vi "Untitled 1.vi"() -> ()   [LabVIEW 2018]
panel:
  out "error out":errorcluster
  out "Image Display":T1(plugin-control)
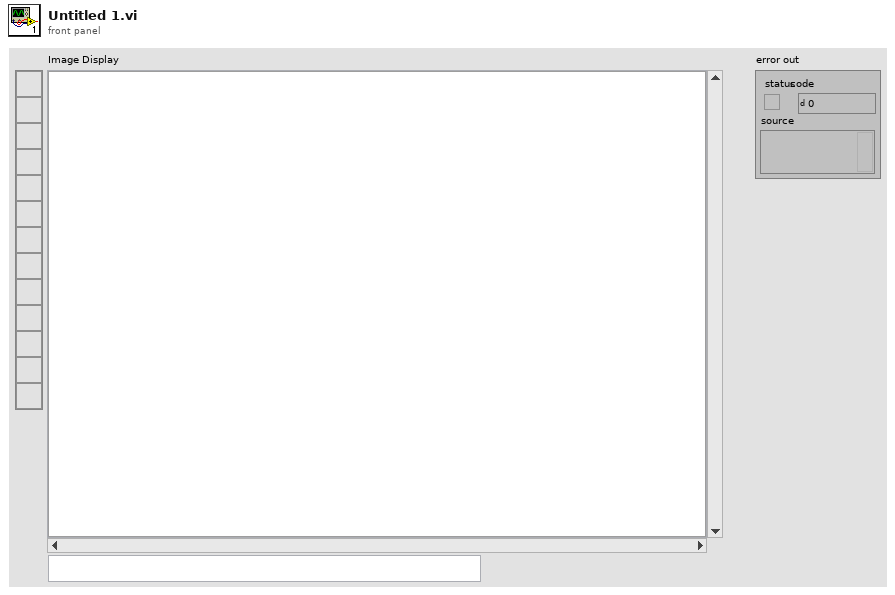
[diagram p1: front panel]
types:
  T1 = typedef "IMAQ Image.ctl" = refnum<image>
  T2 = typedef "Image Type" = u32
  T3 = typedef "imagedata.ctl" = cluster{"image type":i32, "image depth":i32, "image":u8[], "mask":u8[], "colors":u32[], "Rectangle":cluster{"left":i16, "top":i16, "right":i16, "bottom":i16}}
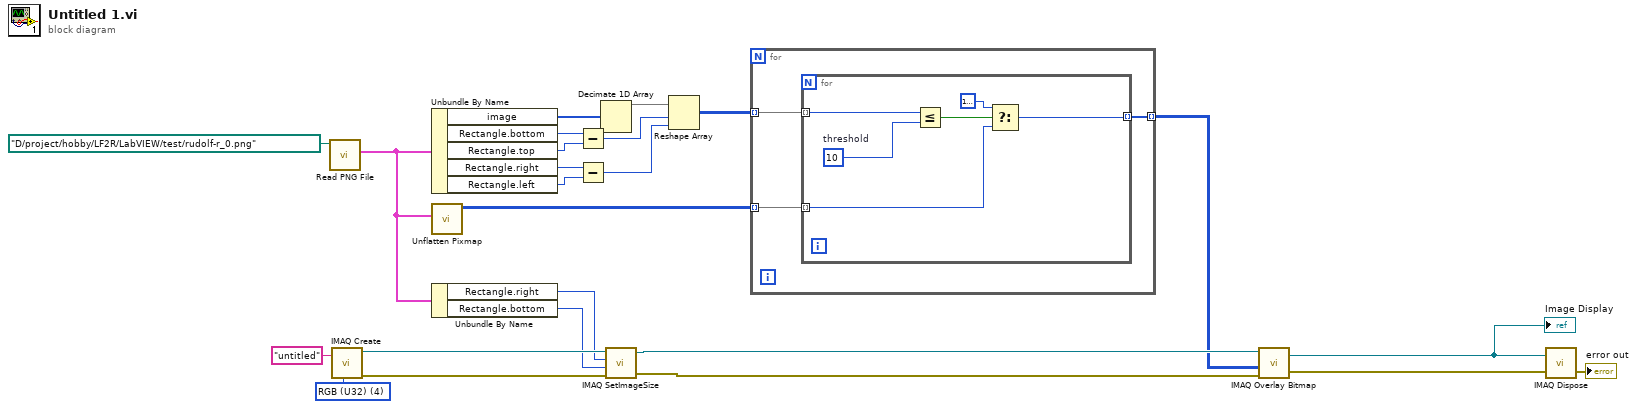
[diagram p0: block diagram]
diagram:
  w23 = T2 4 items=["Grayscale (U8)", "Grayscale (I16)", "Grayscale (SGL)", "Complex (CSG)", "RGB (U32)", "HSL (U32)", "RGB (U64)", "Grayscale (U16)"] ("Image Type")
  n1 = call <vilib>:"Read PNG File.vi"("path to PNG file"=path "D:/project/hobby/LF2R/LabVIEW/test/rudolf-r_0.png") -> ("image data"=w5:T3)  [unwired: 8 in, 2 out]
  n2 = call "IMAQ Create"("Image Name"="untitled", "Image Type"=w23) -> ("New Image"=w9:T1, "error out"=w8:errorcluster)  [unwired: 3 in]
  n3 = Unbundle By Name(w5) -> ("image"=w17:u8[], "Rectangle.bottom"=w21:i16, "Rectangle.top"=w20:i16, "Rectangle.right"=w19:i16, "Rectangle.left"=w18:i16)
  n4 = call <vilib>:"Unflatten Pixmap.vi"("image data"=w5) -> ("24-bit pixmap"=w2:u32[][])  [unwired: 4 in, 6 out]
  n5 = Unbundle By Name(w5) -> ("Rectangle.right"=w4:i16, "Rectangle.bottom"=w3:i16)
  n6 = Subtract(x=w21, y=w20) -> (x-y=w15:i16)
  n7 = Subtract(x=w19, y=w18) -> (x-y=w14:i16)
  n8 = Decimate 1D Array(w17) -> (w16:u8[])  [unwired: 3 out]
  n9 = call "IMAQ SetImageSize"("error in (no error)"=w8, "Y Resolution"=w3, "X Resolution"=w4, "Image"=w9) -> ("error out"=w7:errorcluster, "Image Out"=w6:T1)  [unwired: 1 in]
  n10 = Reshape Array(w16, w15, w14) -> (w13:u8[][])
  n11 = for {
    tunnel: w13 -> [w27] mode=indexing
    tunnel: w2 -> [w26] mode=indexing
    tunnel: [w25] -> w1 mode=indexing
    n12 = for {
      tunnel: w27 -> [w30] mode=indexing
      tunnel: w26 -> [w32] mode=indexing
      tunnel: [w31] -> w25 mode=indexing
      w28 = u8 10  # threshold
      n13 = Less Or Equal?(x=w30, y=w28) -> (x <= y?=w29:bool)
      n14 = Select(t=u32 16777216, s=w29, f=w32) -> (s? t:f=w31:u32)
    }
  }
  n15 = call "IMAQ Overlay Bitmap"("error in (no error)"=w7, "Bitmap"=w1, "Image"=w6) -> ("error out"=w12:errorcluster, "Image Out"=w11:T1)  [unwired: 7 in]
  "Image Display" <- w11
  n16 = call "IMAQ Dispose"("Image"=w11, "error in (no error)"=w12) -> ("error out"=→"error out":errorcluster)  [unwired: 4 in]
